vi "ATM.vi"() -> ()   [LabVIEW 2018]
doc: "This VI is an ATM with operation Withdraw, Deposit, Balance Enquiry, Transfer Money(to another account)"
panel:
  out "welcome":string
  in  "CARD":bool
  out "Balance":string
  in  "E 3":bool
  in  "E 2":bool
  in  "TRANSFER ACCOUNT NUMBER":string
  in  "E":bool
  out "Message":string
  in  "AMOUNT":string
  in  "Cancel":bool
  in  "SELECT A MODE":T1
  in  "Password":string
  in  "Account Number":string
  in  "Sign_In":bool
  # "ATM"
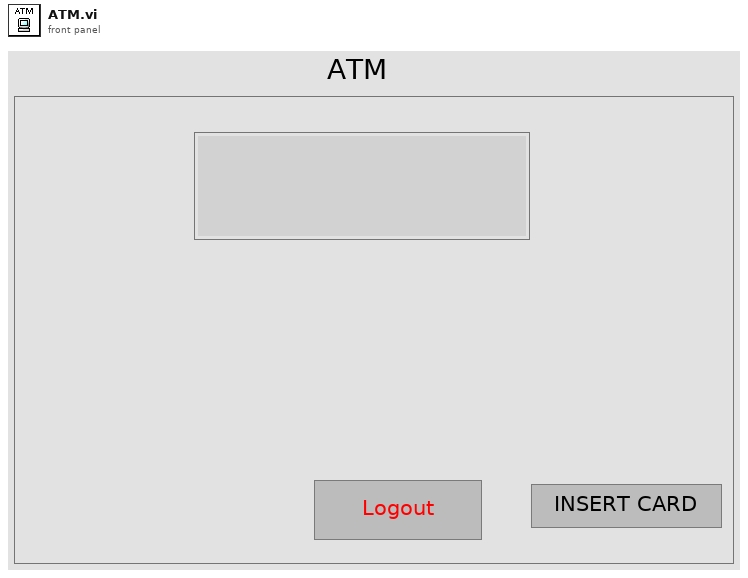
[diagram p1: front panel]
types:
  T1 = cluster{"WITHDRAW":bool, "DEPOSIT":bool, "BALANCE ":bool, "TRANSFER":bool}
  T2 = enum16{"LOGIN", "OPERATION", "WITHDRAW", "DEPOSIT", "BALANCE", "TRANSFER", "LOGOUT"}
  T3 = enum16{"LOGIN", "OPERATION", "WITHDRAW", "DEPOSIT", "BALANCE", "TRANSFER"}
  T4 = enum16{"open", "replace", "create", "open or create", "replace or create", "replace or create with confirmation"}
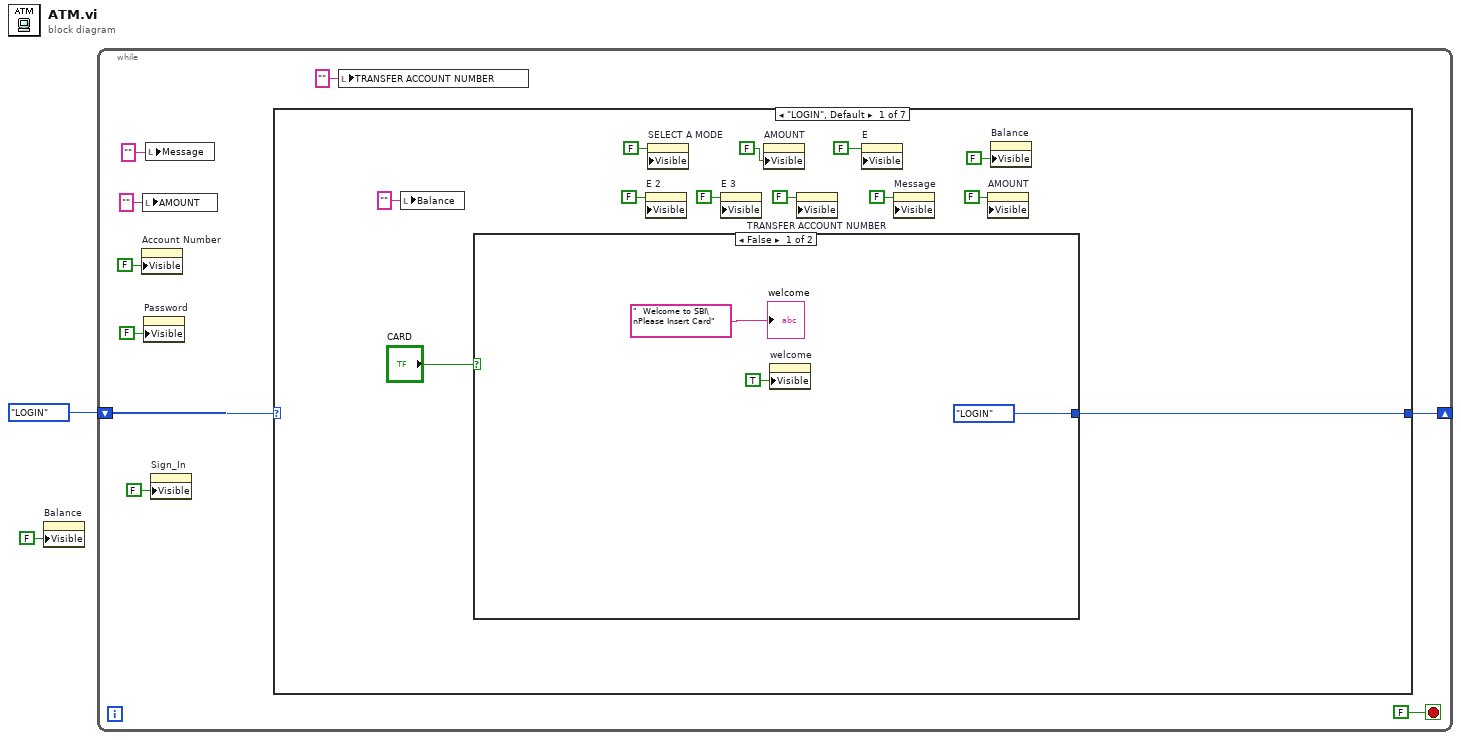
[diagram p0: block diagram]
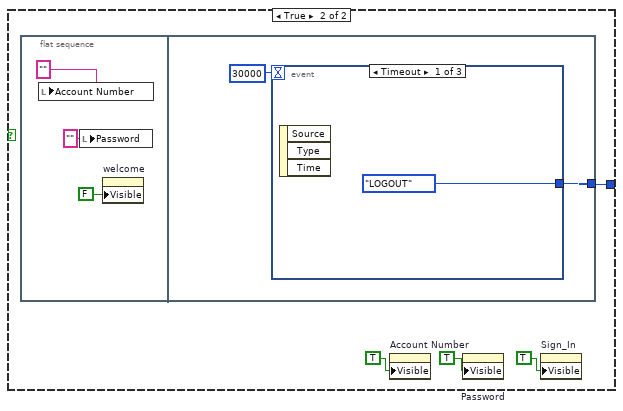
[diagram p2: hidden frame]
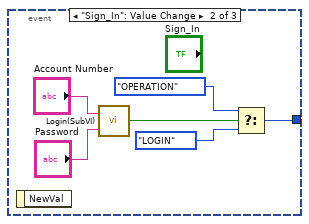
[diagram p3: hidden frame]
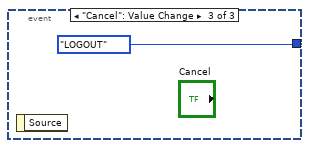
[diagram p4: hidden frame]
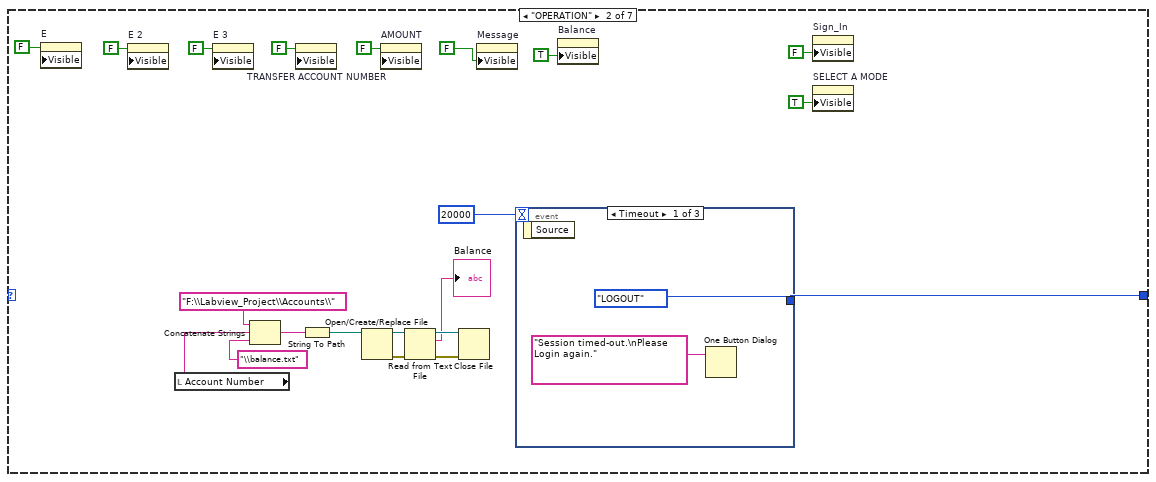
[diagram p5: hidden frame]
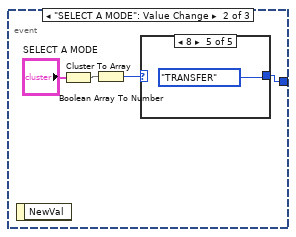
[diagram p6: hidden frame]
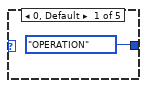
[diagram p7: hidden frame]
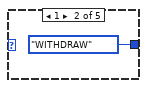
[diagram p8: hidden frame]
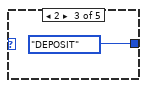
[diagram p9: hidden frame]
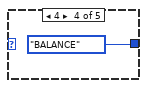
[diagram p10: hidden frame]
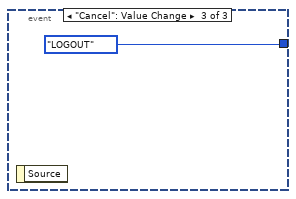
[diagram p11: hidden frame]
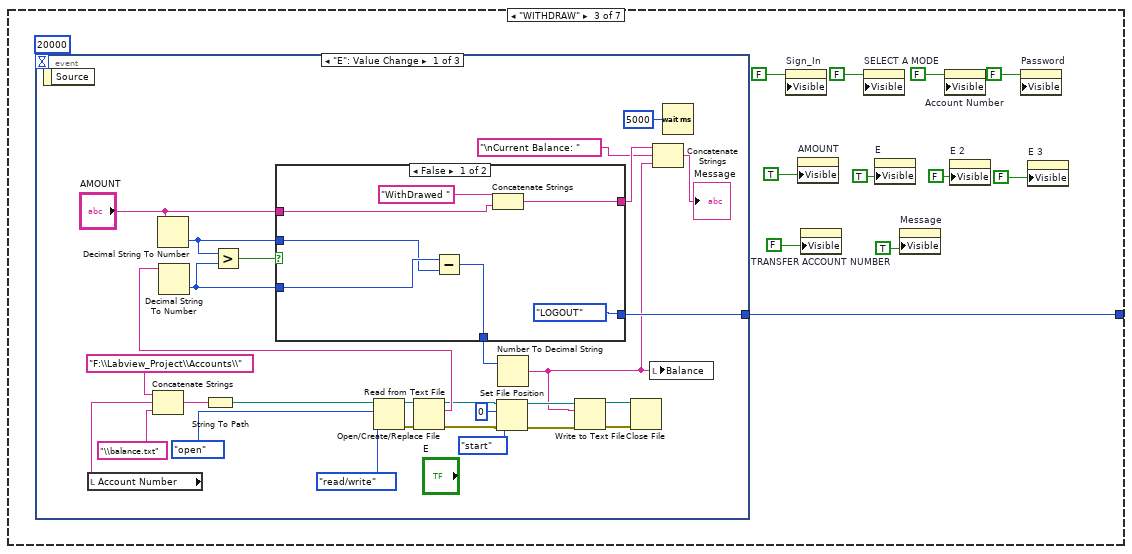
[diagram p12: hidden frame]
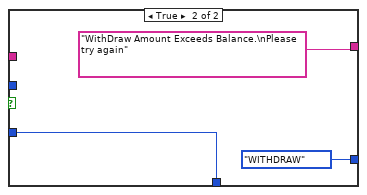
[diagram p13: hidden frame]
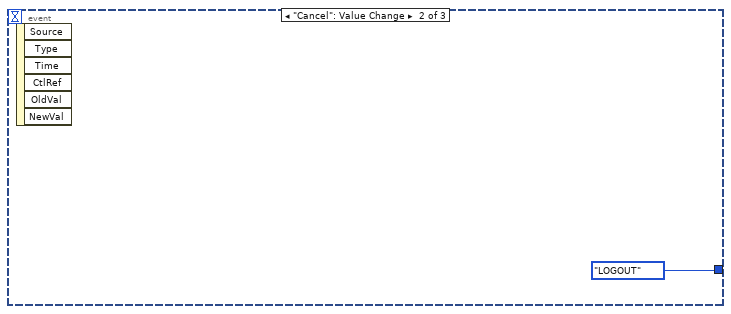
[diagram p14: hidden frame]
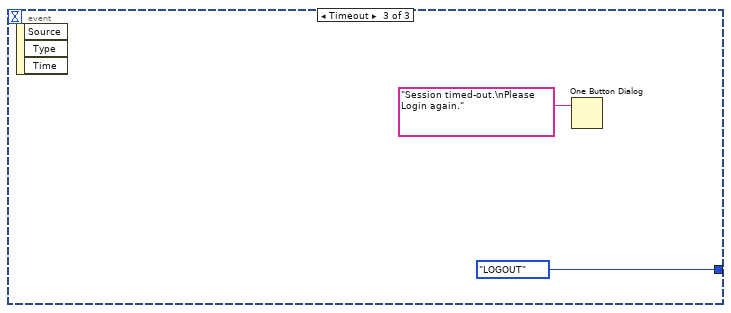
[diagram p15: hidden frame]
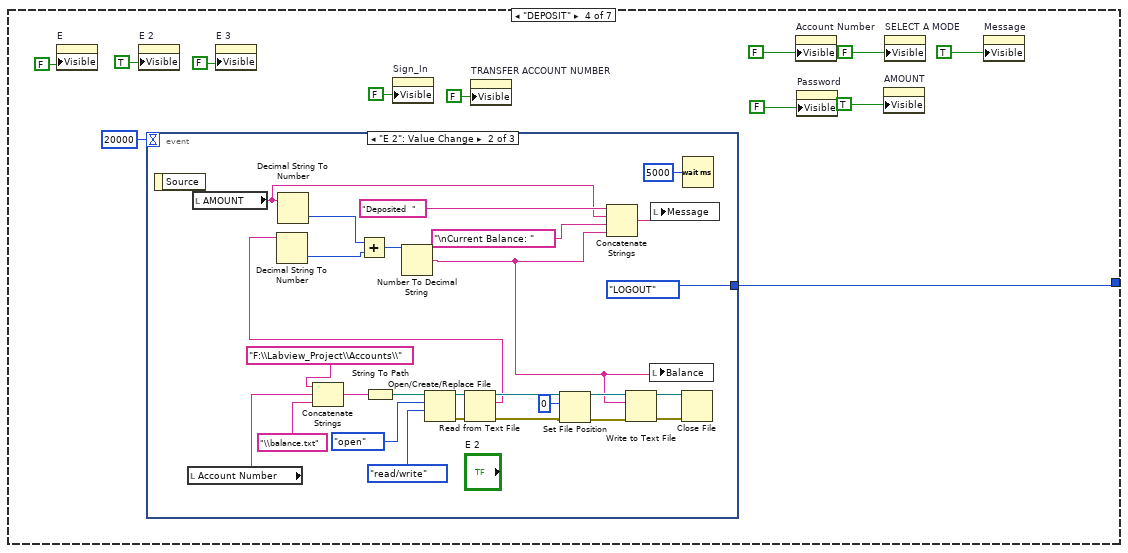
[diagram p16: hidden frame]
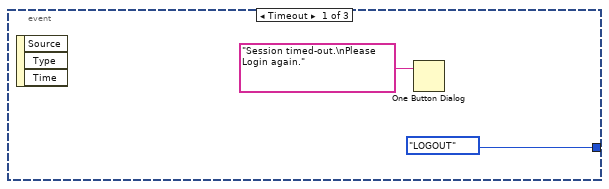
[diagram p17: hidden frame]
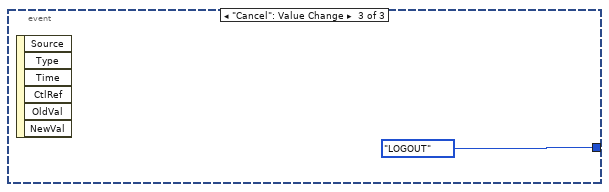
[diagram p18: hidden frame]
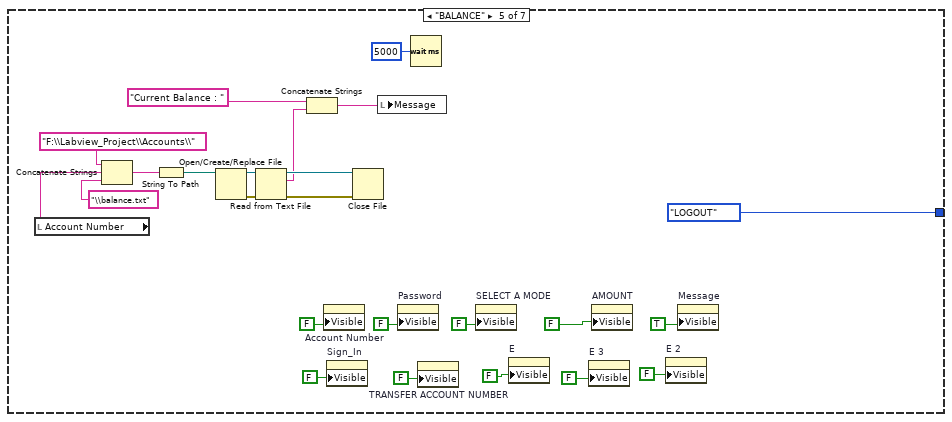
[diagram p19: hidden frame]
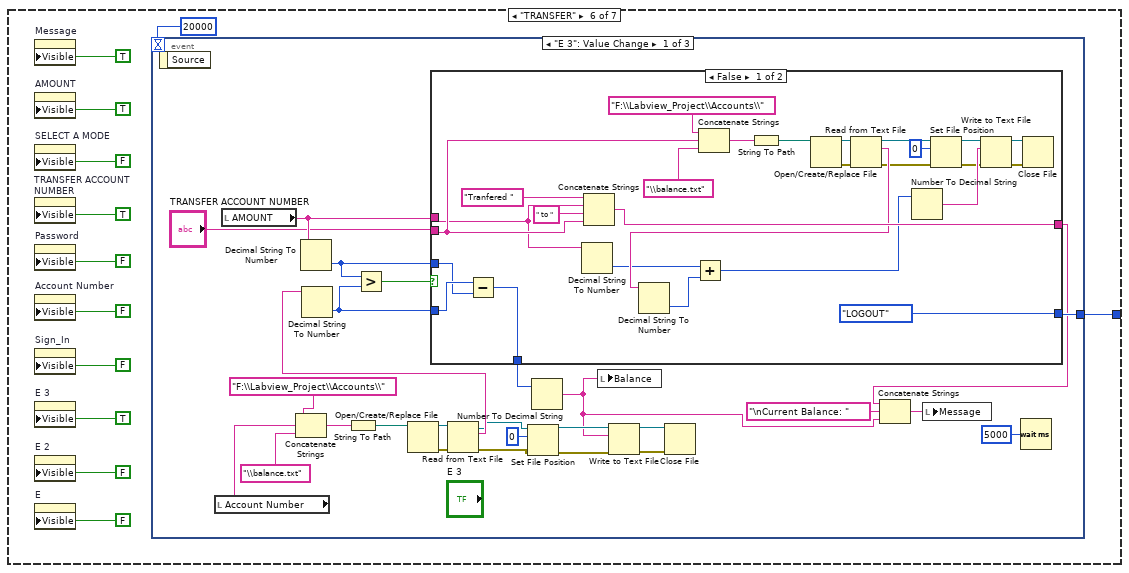
[diagram p20: hidden frame]
diagram:
  n1 = property on="Balance" class="Str"("Visible"=FALSE) -> ()  [unwired: 2 in, 2 out]
  n2 = while {
    shift-right: [w10] -> _
    shift-left: T2."LOGIN" -> [w11]
    stop <- FALSE stop-if-true
    n3 = property on="Account Number" class="Str"("Visible"=FALSE) -> ()  [unwired: 2 in, 2 out]
    n4 = local write "AMOUNT"("" ("AMOUNT")) -> ()
    n5 = property on="Password" class="Str"("Visible"=FALSE) -> ()  [unwired: 2 in, 2 out]
    n6 = local write "Message"("" ("Message")) -> ()
    n7 = property on="Sign_In" class="Bool"("Visible"=FALSE) -> ()  [unwired: 2 in, 2 out]
    n8 = case shown="\"LOGIN\", Default" w11 {
      tunnel: [w23 w64 w88 w142 T2."LOGOUT" w208 T2."LOGOUT"] -> w10
      frame "LOGIN", Default {
        n9 = local write "Balance"("" ("Balance")) -> ()
        n10 = case shown="False" "CARD" {
          tunnel: [T3."LOGIN" w30] -> w23
          frame False {
            n11 = property on="welcome" class="Str"("Visible"=TRUE) -> ()  [unwired: 2 in, 2 out]
            "welcome" <- "  Welcome to SBI\nPlease Insert Card" ("welcome")
          }
          frame True {
            n12 = flat-sequence {
              tunnel: [w34] -> w30
              frame #0 {
                n13 = local write "Account Number"("" ("Account Number")) -> ()
                n14 = local write "Password"("" ("Password")) -> ()
                n15 = property on="welcome" class="Str"("Visible"=FALSE) -> ()  [unwired: 2 in, 2 out]
              }
              frame #1 {
                n16 = event shown="[0] Timeout" {
                  selector: _ -> [_ _ _]
                  dyn-events: _ -> [_ _ _]
                  timeout: 30000 -> [_ _ _]
                  tunnel: [T2."LOGOUT" w37 T2."LOGOUT"] -> w34
                  event Timeout {
                    n17 = event-data() -> ()  [unwired: 1 in, 3 out]
                  }
                  event "Sign_In": Value Change {
                    n18 = event-data() -> ()  [unwired: 1 in, 1 out]
                    n19 = call "Login(SubVI).vi"("Passsword"="Password", "Account"="Account Number") -> ("Status"=w40:bool)
                    n20 = Select(t=T3."OPERATION", s=w40, f=T3."LOGIN") -> (s? t:f=w37:T3)
                  }
                  event "Cancel": Value Change {
                    n21 = event-data() -> ()  [unwired: 1 in, 1 out]
                  }
                }
              }
            }
            n22 = property on="Account Number" class="Str"("Visible"=TRUE) -> ()  [unwired: 2 in, 2 out]
            n23 = property on="Password" class="Str"("Visible"=TRUE) -> ()  [unwired: 2 in, 2 out]
            n24 = property on="Sign_In" class="Bool"("Visible"=TRUE) -> ()  [unwired: 2 in, 2 out]
          }
        }
        n25 = property on="E 2" class="Bool"("Visible"=FALSE) -> ()  [unwired: 2 in, 2 out]
        n26 = property on="SELECT A MODE" class="Clust"("Visible"=FALSE) -> ()  [unwired: 2 in, 2 out]
        n27 = property on="E 3" class="Bool"("Visible"=FALSE) -> ()  [unwired: 2 in, 2 out]
        n28 = property on="AMOUNT" class="Str"("Visible"=FALSE) -> ()  [unwired: 2 in, 2 out]
        n29 = property on="TRANSFER ACCOUNT NUMBER" class="Str"("Visible"=FALSE) -> ()  [unwired: 2 in, 2 out]
        n30 = property on="E" class="Bool"("Visible"=FALSE) -> ()  [unwired: 2 in, 2 out]
        n31 = property on="Message" class="Str"("Visible"=FALSE) -> ()  [unwired: 2 in, 2 out]
        n32 = property on="AMOUNT" class="Str"("Visible"=FALSE) -> ()  [unwired: 2 in, 2 out]
        n33 = property on="Balance" class="Str"("Visible"=FALSE) -> ()  [unwired: 2 in, 2 out]
      }
      frame "OPERATION" {
        n34 = property on="E" class="Bool"("Visible"=FALSE) -> ()  [unwired: 2 in, 2 out]
        n35 = property on="E 2" class="Bool"("Visible"=FALSE) -> ()  [unwired: 2 in, 2 out]
        n36 = local read "Account Number"() -> (w45:string)
        n37 = property on="E 3" class="Bool"("Visible"=FALSE) -> ()  [unwired: 2 in, 2 out]
        n38 = Concatenate Strings("F:\\Labview_Project\\Accounts\\", w45, "\\balance.txt") -> (w51:string)
        n39 = property on="TRANSFER ACCOUNT NUMBER" class="Str"("Visible"=FALSE) -> ()  [unwired: 2 in, 2 out]
        n40 = String To Path(string=w51) -> (path=w52:path)
        n41 = Open/Create/Replace File(file path (use dialog)=w52) -> (refnum out=w54:refnum<file>, error out=w53:errorcluster)  [unwired: 5 in, 1 out]
        n42 = property on="AMOUNT" class="Str"("Visible"=FALSE) -> ()  [unwired: 2 in, 2 out]
        n43 = Read from Text File(file (use dialog)=w54, error in=w53) -> (refnum out=w48:refnum<file>, text=→"Balance":string, error out=w47:errorcluster)  [unwired: 2 in, 1 out]
        n44 = Close File(refnum=w48, error in=w47) -> ()  [unwired: 2 out]
        n45 = property on="Message" class="Str"("Visible"=FALSE) -> ()  [unwired: 2 in, 2 out]
        n46 = event shown="[0] Timeout" {
          selector: _ -> [_ _ _]
          dyn-events: _ -> [_ _ _]
          timeout: 20000 -> [_ _ _]
          tunnel: [T2."LOGOUT" w67 T2."LOGOUT"] -> w64
          event Timeout {
            n47 = event-data() -> ()  [unwired: 1 in, 1 out]
            n48 = One Button Dialog(message="Session timed-out.\nPlease Login again.") -> ()  [unwired: 1 in, 1 out]
          }
          event "SELECT A MODE": Value Change {
            n49 = event-data() -> ()  [unwired: 1 in, 1 out]
            n50 = Cluster To Array(cluster="SELECT A MODE") -> (array=w68:bool[])
            n51 = Boolean Array To Number(Boolean array=w68) -> (number=w70:u32)
            n52 = case shown="8" w70 {
              tunnel: [T3."OPERATION" T3."WITHDRAW" T3."DEPOSIT" T3."BALANCE" T3."TRANSFER"] -> w67
              frame 0, Default {
              }
              frame 1 {
              }
              frame 2 {
              }
              frame 4 {
              }
              frame 8 {
              }
            }
          }
          event "Cancel": Value Change {
            n53 = event-data() -> ()  [unwired: 1 in, 1 out]
          }
        }
        n54 = property on="Balance" class="Str"("Visible"=TRUE) -> ()  [unwired: 2 in, 2 out]
        n55 = property on="Sign_In" class="Bool"("Visible"=FALSE) -> ()  [unwired: 2 in, 2 out]
        n56 = property on="SELECT A MODE" class="Clust"("Visible"=TRUE) -> ()  [unwired: 2 in, 2 out]
      }
      frame "WITHDRAW" {
        n57 = event shown="[0] \"E\": Value Change" {
          selector: _ -> [_ _ _]
          dyn-events: _ -> [_ _ _]
          timeout: 20000 -> [_ _ _]
          tunnel: [w100 T2."LOGOUT" T2."LOGOUT"] -> w88
          event "E": Value Change {
            n58 = event-data() -> ()  [unwired: 1 in, 1 out]
            n59 = local read "Account Number"() -> (w116:string)
            n60 = Concatenate Strings("F:\\Labview_Project\\Accounts\\", w116, "\\balance.txt") -> (w114:string)
            n61 = Decimal String To Number(string="AMOUNT") -> (number=w106:i32)  [unwired: 2 in, 1 out]
            n62 = String To Path(string=w114) -> (path=w113:path)
            n63 = Open/Create/Replace File(file path (use dialog)=w113, operation (0:open)=T4."open", access (0:read/write)=enum16{"read/write", "read-only", "write-only"}."read/write") -> (refnum out=w109:refnum<file>, error out=w110:errorcluster)  [unwired: 3 in, 1 out]
            n64 = Read from Text File(file (use dialog)=w109, error in=w110) -> (refnum out=w97:refnum<file>, text=w108:string, error out=w96:errorcluster)  [unwired: 2 in, 1 out]
            n65 = Decimal String To Number(string=w108) -> (number=w105:i32)  [unwired: 2 in, 1 out]
            n66 = Greater?(x=w106, y=w105) -> (0:w107:bool)
            n67 = case shown="False" w107 {
              tunnel: [T2."LOGOUT" T3."WITHDRAW"] -> w100
              tunnel: w106 -> [w123 _]
              tunnel: w105 -> [w124 w126]
              tunnel: [w122 w126] -> w104
              tunnel: "AMOUNT" -> [w120 _]
              tunnel: [w119 "WithDraw Amount Exceeds Balance.\nPlease try again" ("message")] -> w91
              frame False {
                n68 = Subtract(x=w124, y=w123) -> (x-y=w122:i32)
                n69 = Concatenate Strings("WithDrawed ", w120) -> (w119:string)
              }
              frame True {
              }
            }
            n70 = Set File Position(offset (in bytes) (0)=i64 0, refnum=w97, from (0:start)=enum16{"start", "end", "current"}."start", error in=w96) -> (refnum out=w98:refnum<file>, error out=w95:errorcluster)
            n71 = Number To Decimal String(number=w104) -> (decimal integer string=w89:string)  [unwired: 1 in]
            n72 = Write to Text File(file (use dialog)=w98, text=w89, error in=w95) -> (refnum out=w102:refnum<file>, error out=w103:errorcluster)  [unwired: 1 in, 1 out]
            n73 = Close File(refnum=w102, error in=w103) -> ()  [unwired: 2 out]
            n74 = local write "Balance"(w89) -> ()
            n75 = Concatenate Strings(w91, "\nCurrent Balance: " ("string"), w89) -> (→"Message":string)
            n76 = Wait (ms)(milliseconds to wait=u32 5000) -> ()  [unwired: 1 out]
          }
          event "Cancel": Value Change {
            n77 = event-data() -> ()  [unwired: 1 in, 6 out]
          }
          event Timeout {
            n78 = event-data() -> ()  [unwired: 1 in, 3 out]
            n79 = One Button Dialog(message="Session timed-out.\nPlease Login again.") -> ()  [unwired: 1 in, 1 out]
          }
        }
        n80 = property on="Sign_In" class="Bool"("Visible"=FALSE) -> ()  [unwired: 2 in, 2 out]
        n81 = property on="AMOUNT" class="Str"("Visible"=TRUE) -> ()  [unwired: 2 in, 2 out]
        n82 = property on="TRANSFER ACCOUNT NUMBER" class="Str"("Visible"=FALSE) -> ()  [unwired: 2 in, 2 out]
        n83 = property on="SELECT A MODE" class="Clust"("Visible"=FALSE) -> ()  [unwired: 2 in, 2 out]
        n84 = property on="E" class="Bool"("Visible"=TRUE) -> ()  [unwired: 2 in, 2 out]
        n85 = property on="Message" class="Str"("Visible"=TRUE) -> ()  [unwired: 2 in, 2 out]
        n86 = property on="Account Number" class="Str"("Visible"=FALSE) -> ()  [unwired: 2 in, 2 out]
        n87 = property on="E 2" class="Bool"("Visible"=FALSE) -> ()  [unwired: 2 in, 2 out]
        n88 = property on="Password" class="Str"("Visible"=FALSE) -> ()  [unwired: 2 in, 2 out]
        n89 = property on="E 3" class="Bool"("Visible"=FALSE) -> ()  [unwired: 2 in, 2 out]
      }
      frame "DEPOSIT" {
        n90 = property on="E" class="Bool"("Visible"=FALSE) -> ()  [unwired: 2 in, 2 out]
        n91 = property on="E 2" class="Bool"("Visible"=TRUE) -> ()  [unwired: 2 in, 2 out]
        n92 = event shown="[1] \"E 2\": Value Change" {
          selector: _ -> [_ _ _]
          dyn-events: _ -> [_ _ _]
          timeout: 20000 -> [_ _ _]
          tunnel: [T2."LOGOUT" T2."LOGOUT" T2."LOGOUT"] -> w142
          event Timeout {
            n93 = event-data() -> ()  [unwired: 1 in, 3 out]
            n94 = One Button Dialog(message="Session timed-out.\nPlease Login again.") -> ()  [unwired: 1 in, 1 out]
          }
          event "E 2": Value Change {
            n95 = event-data() -> ()  [unwired: 1 in, 1 out]
            n96 = local read "Account Number"() -> (w171:string)
            n97 = local read "AMOUNT"() -> (w146:string)
            n98 = Decimal String To Number(string=w146) -> (number=w158:i32)  [unwired: 2 in, 1 out]
            n99 = Concatenate Strings("F:\\Labview_Project\\Accounts\\", w171, "\\balance.txt") -> (w165:string)
            n100 = String To Path(string=w165) -> (path=w166:path)
            n101 = Open/Create/Replace File(file path (use dialog)=w166, operation (0:open)=T4."open", access (0:read/write)=enum16{"read/write", "read-only", "write-only"}."read/write") -> (refnum out=w168:refnum<file>, error out=w167:errorcluster)  [unwired: 3 in, 1 out]
            n102 = Read from Text File(file (use dialog)=w168, error in=w167) -> (refnum out=w154:refnum<file>, text=w149:string, error out=w153:errorcluster)  [unwired: 2 in, 1 out]
            n103 = Decimal String To Number(string=w149) -> (number=w150:i32)  [unwired: 2 in, 1 out]
            n104 = Add(x=w158, y=w150) -> (x+y=w157:i32)
            n105 = Number To Decimal String(number=w157) -> (decimal integer string=w147:string)  [unwired: 1 in]
            n106 = Set File Position(offset (in bytes) (0)=i64 0, refnum=w154, error in=w153) -> (refnum out=w151:refnum<file>, error out=w152:errorcluster)  [unwired: 1 in]
            n107 = Concatenate Strings("Deposited  ", w146, "\nCurrent Balance: " ("string"), w147) -> (w160:string)
            n108 = Write to Text File(file (use dialog)=w151, text=w147, error in=w152) -> (refnum out=w170:refnum<file>, error out=w169:errorcluster)  [unwired: 1 in, 1 out]
            n109 = local write "Balance"(w147) -> ()
            n110 = local write "Message"(w160) -> ()
            n111 = Close File(refnum=w170, error in=w169) -> ()  [unwired: 2 out]
            n112 = Wait (ms)(milliseconds to wait=u32 5000) -> ()  [unwired: 1 out]
          }
          event "Cancel": Value Change {
            n113 = event-data() -> ()  [unwired: 1 in, 6 out]
          }
        }
        n114 = property on="E 3" class="Bool"("Visible"=FALSE) -> ()  [unwired: 2 in, 2 out]
        n115 = property on="Sign_In" class="Bool"("Visible"=FALSE) -> ()  [unwired: 2 in, 2 out]
        n116 = property on="TRANSFER ACCOUNT NUMBER" class="Str"("Visible"=FALSE) -> ()  [unwired: 2 in, 2 out]
        n117 = property on="Account Number" class="Str"("Visible"=FALSE) -> ()  [unwired: 2 in, 2 out]
        n118 = property on="Password" class="Str"("Visible"=FALSE) -> ()  [unwired: 2 in, 2 out]
        n119 = property on="AMOUNT" class="Str"("Visible"=TRUE) -> ()  [unwired: 2 in, 2 out]
        n120 = property on="SELECT A MODE" class="Clust"("Visible"=FALSE) -> ()  [unwired: 2 in, 2 out]
        n121 = property on="Message" class="Str"("Visible"=TRUE) -> ()  [unwired: 2 in, 2 out]
      }
      frame "BALANCE" {
        n122 = local read "Account Number"() -> (w196:string)
        n123 = Concatenate Strings("F:\\Labview_Project\\Accounts\\", w196, "\\balance.txt") -> (w192:string)
        n124 = String To Path(string=w192) -> (path=w193:path)
        n125 = Open/Create/Replace File(file path (use dialog)=w193) -> (refnum out=w195:refnum<file>, error out=w194:errorcluster)  [unwired: 5 in, 1 out]
        n126 = Read from Text File(file (use dialog)=w195, error in=w194) -> (refnum out=w189:refnum<file>, text=w186:string, error out=w188:errorcluster)  [unwired: 2 in, 1 out]
        n127 = Concatenate Strings("Current Balance : " ("string"), w186) -> (w185:string)
        n128 = property on="Account Number" class="Str"("Visible"=FALSE) -> ()  [unwired: 2 in, 2 out]
        n129 = property on="Sign_In" class="Bool"("Visible"=FALSE) -> ()  [unwired: 2 in, 2 out]
        n130 = Close File(refnum=w189, error in=w188) -> ()  [unwired: 2 out]
        n131 = local write "Message"(w185) -> ()
        n132 = property on="Password" class="Str"("Visible"=FALSE) -> ()  [unwired: 2 in, 2 out]
        n133 = Wait (ms)(milliseconds to wait=u32 5000) -> ()  [unwired: 1 out]
        n134 = property on="TRANSFER ACCOUNT NUMBER" class="Str"("Visible"=FALSE) -> ()  [unwired: 2 in, 2 out]
        n135 = property on="SELECT A MODE" class="Clust"("Visible"=FALSE) -> ()  [unwired: 2 in, 2 out]
        n136 = property on="E" class="Bool"("Visible"=FALSE) -> ()  [unwired: 2 in, 2 out]
        n137 = property on="E 3" class="Bool"("Visible"=FALSE) -> ()  [unwired: 2 in, 2 out]
        n138 = property on="AMOUNT" class="Str"("Visible"=FALSE) -> ()  [unwired: 2 in, 2 out]
        n139 = property on="E 2" class="Bool"("Visible"=FALSE) -> ()  [unwired: 2 in, 2 out]
        n140 = property on="Message" class="Str"("Visible"=TRUE) -> ()  [unwired: 2 in, 2 out]
      }
      frame "TRANSFER" {
        n141 = property on="Message" class="Str"("Visible"=TRUE) -> ()  [unwired: 2 in, 2 out]
        n142 = property on="AMOUNT" class="Str"("Visible"=TRUE) -> ()  [unwired: 2 in, 2 out]
        n143 = property on="SELECT A MODE" class="Clust"("Visible"=FALSE) -> ()  [unwired: 2 in, 2 out]
        n144 = property on="TRANSFER ACCOUNT NUMBER" class="Str"("Visible"=TRUE) -> ()  [unwired: 2 in, 2 out]
        n145 = property on="Password" class="Str"("Visible"=FALSE) -> ()  [unwired: 2 in, 2 out]
        n146 = property on="Account Number" class="Str"("Visible"=FALSE) -> ()  [unwired: 2 in, 2 out]
        n147 = property on="Sign_In" class="Bool"("Visible"=FALSE) -> ()  [unwired: 2 in, 2 out]
        n148 = property on="E 3" class="Bool"("Visible"=TRUE) -> ()  [unwired: 2 in, 2 out]
        n149 = property on="E 2" class="Bool"("Visible"=FALSE) -> ()  [unwired: 2 in, 2 out]
        n150 = property on="E" class="Bool"("Visible"=FALSE) -> ()  [unwired: 2 in, 2 out]
        n151 = event shown="[0] \"E 3\": Value Change" {
          selector: _ -> [_ _ _]
          dyn-events: _ -> [_ _ _]
          timeout: 20000 -> [_ _ _]
          tunnel: [w219 T2."LOGOUT" T2."LOGOUT"] -> w208
          event "E 3": Value Change {
            n152 = event-data() -> ()  [unwired: 1 in, 1 out]
            n153 = local read "Account Number"() -> (w235:string)
            n154 = local read "AMOUNT"() -> (w234:string)
            n155 = Concatenate Strings("F:\\Labview_Project\\Accounts\\", w235, "\\balance.txt") -> (w233:string)
            n156 = Decimal String To Number(string=w234) -> (number=w227:i32)  [unwired: 2 in, 1 out]
            n157 = String To Path(string=w233) -> (path=w232:path)
            n158 = Open/Create/Replace File(file path (use dialog)=w232) -> (refnum out=w230:refnum<file>, error out=w231:errorcluster)  [unwired: 5 in, 1 out]
            n159 = Read from Text File(file (use dialog)=w230, error in=w231) -> (refnum out=w213:refnum<file>, text=w229:string, error out=w216:errorcluster)  [unwired: 2 in, 1 out]
            n160 = Decimal String To Number(string=w229) -> (number=w226:i32)  [unwired: 2 in, 1 out]
            n161 = Greater?(x=w227, y=w226) -> (0:w228:bool)
            n162 = case shown="False" w228 {
              tunnel: [T2."LOGOUT" T2."WITHDRAW"] -> w219
              tunnel: w227 -> [w261 _]
              tunnel: w226 -> [w262 w265]
              tunnel: [w260 w265] -> w225
              tunnel: w234 -> [w246 _]
              tunnel: [w258 "WithDraw Amount Exceeds\nBalance. Please try again" ("message")] -> w211
              tunnel: "TRANSFER ACCOUNT NUMBER" -> [w247 _]
              frame False {
                n163 = Subtract(x=w262, y=w261) -> (x-y=w260:i32)
                n164 = Decimal String To Number(string=w246) -> (number=w244:i32)  [unwired: 2 in, 1 out]
                n165 = Concatenate Strings("Tranfered ", w246, " to " ("string"), w247) -> (w258:string)
                n166 = Concatenate Strings("F:\\Labview_Project\\Accounts\\", w247, "\\balance.txt") -> (w250:string)
                n167 = String To Path(string=w250) -> (path=w251:path)
                n168 = Open/Create/Replace File(file path (use dialog)=w251) -> (refnum out=w253:refnum<file>, error out=w252:errorcluster)  [unwired: 5 in, 1 out]
                n169 = Read from Text File(file (use dialog)=w253, error in=w252) -> (refnum out=w241:refnum<file>, text=w245:string, error out=w238:errorcluster)  [unwired: 2 in, 1 out]
                n170 = Decimal String To Number(string=w245) -> (number=w237:i32)  [unwired: 2 in, 1 out]
                n171 = Add(x=w244, y=w237) -> (x+y=w243:i32)
                n172 = Number To Decimal String(number=w243) -> (decimal integer string=w254:string)  [unwired: 1 in]
                n173 = Set File Position(offset (in bytes) (0)=i64 0, refnum=w241, error in=w238) -> (refnum out=w240:refnum<file>, error out=w239:errorcluster)  [unwired: 1 in]
                n174 = Write to Text File(file (use dialog)=w240, text=w254, error in=w239) -> (refnum out=w256:refnum<file>, error out=w255:errorcluster)  [unwired: 1 in, 1 out]
                n175 = Close File(refnum=w256, error in=w255) -> ()  [unwired: 2 out]
              }
              frame True {
              }
            }
            n176 = Set File Position(offset (in bytes) (0)=i64 0, refnum=w213, error in=w216) -> (refnum out=w214:refnum<file>, error out=w215:errorcluster)  [unwired: 1 in]
            n177 = Number To Decimal String(number=w225) -> (decimal integer string=w210:string)  [unwired: 1 in]
            n178 = local write "Balance"(w210) -> ()
            n179 = Write to Text File(file (use dialog)=w214, text=w210, error in=w215) -> (refnum out=w223:refnum<file>, error out=w224:errorcluster)  [unwired: 1 in, 1 out]
            n180 = Close File(refnum=w223, error in=w224) -> ()  [unwired: 2 out]
            n181 = Concatenate Strings(w211, "\nCurrent Balance: " ("string"), w210) -> (w209:string)
            n182 = local write "Message"(w209) -> ()
            n183 = Wait (ms)(milliseconds to wait=u32 5000) -> ()  [unwired: 1 out]
          }
          event "Cancel": Value Change {
            n184 = event-data() -> ()  [unwired: 1 in, 6 out]
          }
          event Timeout {
            n185 = event-data() -> ()  [unwired: 1 in, 3 out]
            n186 = One Button Dialog(message="Session timed-out.\nPlease Login again.") -> ()  [unwired: 1 in, 1 out]
          }
        }
      }
      frame "LOGOUT" {
        w270 = FALSE
        n187 = property on="Message" class="Str"("Visible"=TRUE) -> ()  [unwired: 2 in, 2 out]
        n188 = property on="E 2" class="Bool"("Visible"=w270) -> ()  [unwired: 2 in, 2 out]
        n189 = property on="TRANSFER ACCOUNT NUMBER" class="Str"("Visible"=w270) -> ()  [unwired: 2 in, 2 out]
        n190 = property on="SELECT A MODE" class="Clust"("Visible"=w270) -> ()  [unwired: 2 in, 2 out]
        n191 = property on="E 3" class="Bool"("Visible"=w270) -> ()  [unwired: 2 in, 2 out]
        n192 = property on="Sign_In" class="Bool"("Visible"=w270) -> ()  [unwired: 2 in, 2 out]
        n193 = property on="AMOUNT" class="Str"("Visible"=w270) -> ()  [unwired: 2 in, 2 out]
        n194 = property on="Balance" class="Str"("Visible"=w270) -> ()  [unwired: 2 in, 2 out]
        n195 = property on="E" class="Bool"("Visible"=w270) -> ()  [unwired: 2 in, 2 out]
        n196 = local write "Message"("THANK YOU\nPLEASE COME AGAIN" ("Message")) -> ()
      }
    }
    n197 = local write "TRANSFER ACCOUNT NUMBER"("" ("TRANSFER ACCOUNT NUMBER")) -> ()
  }
